vi "Shock&Dyanamics Laboratory - DROPBEAR_June2022_Rev3.vi"() -> ()   [LabVIEW 2019] (continued)
  in  "PF Card 1":dbl caption="Card" min=0.0 max=7.0 step=1.0 format="%0#2.1g"
  in  "PF Channel 1":dbl=1.0 caption="Channel" min=0.0 max=7.0 step=1.0 format="%0#2.1g"
  out "LED Enable Ch 1":bool=TRUE
  in  "SG Pair Ch 1":T10(ring)=enum."Ch 2"
  in  "SG Pair 2":bool caption="Paired"
  in  "Sens Fac 2":enum16{"uV/MU", "mV/MU", "V/MU"}(ring)=enum."mV/MU"
  in  "PF Condition 2":bool caption="PF Condition"
  in  "PF Chassis 2":dbl caption="Chassis" min=0.0 max=7.0 step=1.0 format="%0#2.1g"
  in  "PF Card 2":dbl caption="Card" min=0.0 max=7.0 step=1.0 format="%0#2.1g"
  in  "PF Channel 2":dbl caption="Channel" min=0.0 max=7.0 step=1.0 format="%0#2.1g"
  in  "Voltage Max Ch 2":dbl=10.0 caption="Max Value"
  in  "Voltage Min Ch 2":dbl=-10.0 caption="Min Value"
  in  "Enable Ch 2":bool=TRUE
  in  "Name Ch 2":string="SG_306_b"
  in  "Physical Channel Ch 2":tag="PXI1Slot5/ai1" caption="Physical Channels"
  in  "Sensitivity 2":dbl=50.0 caption="Sensitivity 0"
  out "LED Enable Ch 2":bool=TRUE
  in  "Signal Type 2":T8(ring)=enum."Strain" caption="Signal Type"
  in  "SG Pair Ch 2":T11(ring)=enum."Unpaired"
  in  "SG Pair 3":bool caption="Paired"
  in  "Sens Fac 3":enum16{"uV/MU", "mV/MU", "V/MU"}(ring)=enum."V/MU"
  in  "PF Condition 3":bool caption="PF Condition"
  in  "PF Chassis 3":dbl caption="Chassis" min=0.0 max=7.0 step=1.0 format="%0#2.1g"
  in  "PF Card 3":dbl caption="Card" min=0.0 max=7.0 step=1.0 format="%0#2.1g"
  in  "PF Channel 3":dbl=1.0 caption="Channel" min=0.0 max=7.0 step=1.0 format="%0#2.1g"
  in  "Voltage Max Ch 3":dbl=10.0 caption="Max Value"
  in  "Voltage Min Ch 3":dbl=-10.0 caption="Min Value"
  in  "Enable Ch 3":bool=TRUE
  in  "Name Ch 3":string="Accel"
  in  "Physical Channels Ch 3":tag="PXI1Slot5/ai4" caption="Physical Channels"
  in  "Sensitivity 3":dbl=2.0 caption="Sensitivity 0"
  out "LED Enable Ch 3":bool=TRUE
  in  "Signal Type 3":T8(ring) caption="Signal Type"
  in  "SG Pair Ch 3":T12(ring)=enum."Unpaired"
  in  "SG Pair 4":bool=TRUE caption="Paired"
  in  "Sens Fac 4":enum16{"uV/MU", "mV/MU", "V/MU"}(ring)=enum."mV/MU"
  in  "PF Condition 4":bool=TRUE caption="PF Condition"
  in  "PF Chassis 4":dbl caption="Chassis" min=0.0 max=7.0 step=1.0 format="%0#2.1g"
  in  "PF Card 4":dbl caption="Card" min=0.0 max=7.0 step=1.0 format="%0#2.1g"
  in  "PF Channel 4":dbl=2.0 caption="Channel" min=0.0 max=7.0 step=1.0 format="%0#2.1g"
  in  "Physical Channel Ch 4":tag="PXI1Slot5/ai5" caption="Physical Channels"
  in  "Name Ch 4":string="LowG_accel"
  in  "Enable Ch 4":bool
  in  "Voltage Max Ch 4":dbl=10.0 caption="Max Value"
  in  "Voltage Min Ch 4":dbl=-10.0 caption="Min Value"
  in  "Sensitivity 4":dbl=1.0 caption="Sensitivity 0"
  out "LED Enable Ch 4":bool
  in  "Signal Type 4":T8(ring)=enum."Voltage" caption="Signal Type"
  in  "SG Pair Ch 4":T13(ring)=enum."Unpaired"
  in  "SG Pair 5":bool=TRUE caption="Paired"
  in  "Sens Fac 5":enum16{"uV/MU", "mV/MU", "V/MU"}(ring)=enum."mV/MU"
  in  "Name Ch 5":string="MassDrop"
  in  "Physical Channel Ch 5":tag="PXI1Slot7/ai0" caption="Physical Channels"
  in  "Enable Ch 5":bool
  in  "Voltage Min Ch 5":dbl=-10.0 caption="Min Value"
  in  "Voltage Max Ch 5":dbl=10.0 caption="Max Value"
  in  "Sensitivity 5":dbl=1.0 caption="Sensitivity 0"
  out "LED Enable Ch 5":bool=TRUE
  in  "Signal Type 5":T8(ring)=enum."Voltage" caption="Signal Type"
  in  "PF Channel 5":dbl=3.0 caption="Channel" min=0.0 max=7.0 step=1.0 format="%0#2.1g"
  in  "PF Card 5":dbl caption="Card" min=0.0 max=7.0 step=1.0 format="%0#2.1g"
  in  "PF Chassis 5":dbl caption="Chassis" min=0.0 max=7.0 step=1.0 format="%0#2.1g"
  in  "PF Condition 5":bool=TRUE caption="PF Condition"
  in  "SG Pair Ch 5":T14(ring)=enum."Unpaired"
  in  "SG Pair 6":bool caption="Paired"
  in  "Sens Fac 6":enum16{"uV/MU", "mV/MU", "V/MU"}(ring)=enum."mV/MU"
  in  "Enable Ch 6":bool=TRUE
  in  "Physical Channels Ch 6":tag="PXI1Slot6/ai0" caption="Physical Channels"
  in  "Voltage Max  Ch 6":dbl=10.0 caption="Max Value"
  in  "Voltage Min Ch 6":dbl=-10.0 caption="Min Value"
  in  "Name Ch 6":string="PinLoc"
  in  "Sensitivity 6":dbl=1.0 caption="Sensitivity 0"
  out "LED Enable Ch 6":bool=TRUE
  in  "Signal Type 6":T8(ring)=enum."Voltage" caption="Signal Type"
  in  "PF Channel 6":dbl caption="Channel" min=0.0 max=7.0 step=1.0 format="%0#2.1g"
  in  "PF Card 6":dbl caption="Card" min=0.0 max=7.0 step=1.0 format="%0#2.1g"
  in  "PF Chassis 6":dbl caption="Chassis" min=0.0 max=7.0 step=1.0 format="%0#2.1g"
  in  "PF Condition 6":bool=TRUE caption="PF Condition"
  in  "SG Pair Ch 6":T15(ring)=enum."Unpaired"
  in  "SG Pair 7":bool=TRUE caption="Paired"
  in  "Sens Fac 7":enum16{"uV/MU", "mV/MU", "V/MU"}(ring)=enum."mV/MU"
  in  "PF Channel 7":dbl=1.0 caption="Channel" min=0.0 max=7.0 step=1.0 format="%0#2.1g"
  in  "PF Card 7":dbl caption="Card" min=0.0 max=7.0 step=1.0 format="%0#2.1g"
  in  "PF Chassis 7":dbl caption="Chassis" min=0.0 max=7.0 step=1.0 format="%0#2.1g"
  in  "PF Condition 7":bool=TRUE caption="PF Condition"
  in  "Enable Ch 7":bool=TRUE
  in  "Physical Channel Ch 7":tag="PXI1Slot7/ai3" caption="Physical Channels"
  in  "Voltage Max Ch 7":dbl=10.0 caption="Max Value"
  in  "Voltage Min Ch 7":dbl=-1.0 caption="Min Value"
  in  "Name Ch 7":string="Extensometer"
  in  "Sensitivity 7":dbl=1.0 caption="Sensitivity 0"
  out "LED Enable Ch 7":bool=TRUE
  in  "Signal Type 7":T8(ring)=enum."Voltage" caption="Signal Type"
  in  "SG Pair Ch 7":T16(ring)=enum."Unpaired"
  in  "SG Pair 8":bool=TRUE caption="Paired"
  in  "Sens Fac 8":enum16{"uV/MU", "mV/MU", "V/MU"}(ring)=enum."mV/MU"
  in  "Enable Ch 8":bool
  in  "Physical Channel Ch 8":tag="PXI1Slot7/ai2" caption="Physical Channels"
  in  "Voltage Max Ch 8":dbl=10.0 caption="Max Value"
  in  "Voltage Min Ch 8":dbl=-10.0 caption="Min Value"
  in  "Name Ch 8":string="StrainGauge_08_000"
  in  "Sensitivity 8":dbl=1.0 caption="Sensitivity 0"
  out "LED Enable Ch 8":bool
  in  "Signal Type 8":T8(ring)=enum."Strain" caption="Signal Type"
  in  "PF Condition 8":bool=TRUE caption="PF Condition"
  in  "PF Chassis 8":dbl caption="Chassis" min=0.0 max=7.0 step=1.0 format="%0#2.1g"
  in  "PF Card 8":dbl caption="Card" min=0.0 max=7.0 step=1.0 format="%0#2.1g"
  in  "PF Channel 8":dbl=2.0 caption="Channel" min=0.0 max=7.0 step=1.0 format="%0#2.1g"
  in  "SG Pair Ch 8":T17(ring)=enum."Unpaired"
  in  "SG Pair 9":bool=TRUE caption="Paired"
  in  "Sens Fac 9":enum16{"uV/MU", "mV/MU", "V/MU"}(ring)=enum."mV/MU"
  in  "PF Condition 9":bool=TRUE caption="PF Condition"
  in  "PF Chassis 9":dbl caption="Chassis" min=0.0 max=7.0 step=1.0 format="%0#2.1g"
  in  "PF Card 9":dbl caption="Card" min=0.0 max=7.0 step=1.0 format="%0#2.1g"
  in  "PF Channel 9":dbl=3.0 caption="Channel" min=0.0 max=7.0 step=1.0 format="%0#2.1g"
  in  "Enable Ch 9":bool
  in  "Physical Channel Ch 9":tag="PXI1Slot7/ai3" caption="Physical Channels"
  in  "Voltage Max Ch 9":dbl=10.0 caption="Max Value"
  in  "Voltage Min Ch 9":dbl=-10.0 caption="Min Value"
  in  "Name Ch 9":string="StrainGauge_08_180"
  in  "Sensitivity 9":dbl=1.0 caption="Sensitivity 0"
  out "LED Enable Ch 9":bool
  in  "Signal Type 9":T8(ring)=enum."Strain" caption="Signal Type"
  in  "SG Pair Ch 9":T18(ring)=enum."Unpaired"
  in  "SG Pair 10":bool=TRUE caption="Paired"
  in  "Sens Fac 10":enum16{"uV/MU", "mV/MU", "V/MU"}(ring)
  in  "PF Condition 10":bool caption="PF Condition"
  in  "PF Chassis 10":dbl caption="Chassis" min=0.0 max=7.0 step=1.0 format="%0#2.1g"
  in  "PF Card 10":dbl caption="Card" min=0.0 max=7.0 step=1.0 format="%0#2.1g"
  in  "PF Channel 10":dbl caption="Channel" min=0.0 max=7.0 step=1.0 format="%0#2.1g"
  in  "Enable Ch 10":bool
  in  "Physical Channel Ch 10":tag="PXI1Slot5/ai2" caption="Physical Channels"
  in  "Voltage Max Ch 10":dbl=10.0 caption="Max Value"
  in  "Voltage Min Ch 10":dbl=-10.0 caption="Min Value"
  in  "Name Ch 10":string="noname"
  in  "Sensitivity 10":dbl=0.2 caption="Sensitivity 0"
  out "LED Enable Ch 10":bool
  in  "Signal Type 10":T8(ring)=enum."Strain" caption="Signal Type"
  in  "SG Pair Ch 10":T19(ring)=enum."Unpaired"
  in  "SG Pair 11":bool=TRUE caption="Paired"
  in  "Sens Fac 11":enum16{"uV/MU", "mV/MU", "V/MU"}(ring)
  in  "PF Condition 11":bool caption="PF Condition"
  in  "PF Chassis 11":dbl caption="Chassis" min=0.0 max=7.0 step=1.0 format="%0#2.1g"
  in  "PF Card 11":dbl caption="Card" min=0.0 max=7.0 step=1.0 format="%0#2.1g"
  in  "PF Channel 11":dbl caption="Channel" min=0.0 max=7.0 step=1.0 format="%0#2.1g"
  in  "Enable Ch 11":bool
  in  "Physical Channel Ch 11":tag="PXI1Slot5/ai2" caption="Physical Channels"
  in  "Voltage Max Ch 11":dbl=10.0 caption="Max Value"
  in  "Voltage Min Ch 11":dbl=-10.0 caption="Min Value"
  in  "Name Ch 11":string="noname"
  in  "Sensitivity 11":dbl=0.2 caption="Sensitivity 0"
  out "LED Enable Ch 11":bool
  in  "Signal Type 11":T8(ring)=enum."Strain" caption="Signal Type"
  in  "SG Pair Ch 11":T20(ring)=enum."Unpaired"
  in  "SG Pair 12":bool=TRUE caption="Paired"
  in  "Sens Fac 12":enum16{"uV/MU", "mV/MU", "V/MU"}(ring)
  in  "PF Condition 12":bool caption="PF Condition"
  in  "PF Chassis 12":dbl caption="Chassis" min=0.0 max=7.0 step=1.0 format="%0#2.1g"
  in  "PF Card 12":dbl caption="Card" min=0.0 max=7.0 step=1.0 format="%0#2.1g"
  in  "PF Channel 12":dbl caption="Channel" min=0.0 max=7.0 step=1.0 format="%0#2.1g"
  in  "Enable Ch 12":bool
  in  "Physical Channel Ch 12":tag="PXI1Slot5/ai2" caption="Physical Channels"
  in  "Voltage Max Ch 12":dbl=10.0 caption="Max Value"
  in  "Voltage Min Ch 12":dbl=-10.0 caption="Min Value"
  in  "Name Ch 12":string="noname"
  in  "Sensitivity 12":dbl=0.2 caption="Sensitivity 0"
  out "LED Enable Ch 12":bool
  in  "Signal Type 12":T8(ring)=enum."Strain" caption="Signal Type"
  in  "SG Pair Ch 12":T21(ring)=enum."Unpaired"
  in  "SG Pair 13":bool=TRUE caption="Paired"
  in  "Sens Fac 13":enum16{"uV/MU", "mV/MU", "V/MU"}(ring)
  in  "PF Condition 13":bool caption="PF Condition"
  in  "PF Chassis 13":dbl caption="Chassis" min=0.0 max=7.0 step=1.0 format="%0#2.1g"
  in  "PF Card 13":dbl caption="Card" min=0.0 max=7.0 step=1.0 format="%0#2.1g"
  in  "PF Channel 13":dbl caption="Channel" min=0.0 max=7.0 step=1.0 format="%0#2.1g"
  in  "Enable Ch 13":bool
  in  "Physical Channel Ch 13":tag="PXI1Slot5/ai2" caption="Physical Channels"
  in  "Voltage Max Ch 13":dbl=10.0 caption="Max Value"
  in  "Voltage Min Ch 13":dbl=-10.0 caption="Min Value"
  in  "Name Ch 13":string="noname"
  in  "Sensitivity 13":dbl=0.2 caption="Sensitivity 0"
  out "LED Enable Ch 13":bool
  in  "Signal Type 13":T8(ring)=enum."Strain" caption="Signal Type"
  in  "SG Pair Ch 13":T22(ring)=enum."Unpaired"
  in  "SG Pair 14":bool=TRUE caption="Paired"
  in  "Sens Fac 14":enum16{"uV/MU", "mV/MU", "V/MU"}(ring)
  in  "PF Condition 14":bool caption="PF Condition"
  in  "PF Chassis 14":dbl caption="Chassis" min=0.0 max=7.0 step=1.0 format="%0#2.1g"
  in  "PF Card 14":dbl caption="Card" min=0.0 max=7.0 step=1.0 format="%0#2.1g"
  in  "PF Channel 14":dbl caption="Channel" min=0.0 max=7.0 step=1.0 format="%0#2.1g"
  in  "Enable Ch 14":bool
  in  "Physical Channel Ch 14":tag="PXI1Slot5/ai2" caption="Physical Channels"
  in  "Voltage Max Ch 14":dbl=10.0 caption="Max Value"
  in  "Voltage Min Ch 14":dbl=-10.0 caption="Min Value"
  in  "Name Ch 14":string="noname"
  in  "Sensitivity 14":dbl=0.2 caption="Sensitivity 0"
  out "LED Enable Ch 14":bool
  in  "Signal Type 14":T8(ring)=enum."Strain" caption="Signal Type"
  in  "SG Pair Ch 14":T23(ring)=enum."Unpaired"
  in  "SG Pair 15":bool=TRUE caption="Paired"
  in  "Sens Fac 15":enum16{"uV/MU", "mV/MU", "V/MU"}(ring)
  in  "PF Condition 15":bool caption="PF Condition"
  in  "PF Chassis 15":dbl caption="Chassis" min=0.0 max=7.0 step=1.0 format="%0#2.1g"
  in  "PF Card 15":dbl caption="Card" min=0.0 max=7.0 step=1.0 format="%0#2.1g"
  in  "PF Channel 15":dbl caption="Channel" min=0.0 max=7.0 step=1.0 format="%0#2.1g"
  in  "Enable Ch 15":bool
  in  "Physical Channel Ch 15":tag="PXI1Slot5/ai2" caption="Physical Channels"
  in  "Voltage Max Ch 15":dbl=10.0 caption="Max Value"
  in  "Voltage Min Ch 15":dbl=-10.0 caption="Min Value"
  in  "Name Ch 15":string="noname"
  in  "Sensitivity 15":dbl=0.2 caption="Sensitivity 0"
  out "LED Enable Ch 15":bool
  in  "Signal Type 15":T8(ring)=enum."Strain" caption="Signal Type"
  in  "SG Pair Ch 15":T24(ring)=enum."Unpaired"
  in  "Enable Ch 16":bool
  in  "Name Ch 16":string="noname"
  in  "Physical Channel Ch 16":tag="PXI1Slot8/ai3" caption="Physical Channels"
  in  "PF Chassis 16":dbl caption="Chassis" min=0.0 max=7.0 step=1.0 format="%0#2.1g"
  in  "PF Card 16":dbl=5.0 caption="Card" min=0.0 max=7.0 step=1.0 format="%0#2.1g"
  in  "PF Channel 16":dbl=3.0 caption="Channel" min=0.0 max=7.0 step=1.0 format="%0#2.1g"
  in  "PF Condition 16":bool=TRUE caption="PF Condition"
  in  "Signal Type 16":T8(ring)=enum."Strain" caption="Signal Type"
  in  "Voltage Max Ch 16":dbl=10.0 caption="Max Value"
  in  "Voltage Min Ch 16":dbl=-10.0 caption="Min Value"
  in  "Sensitivity 16":dbl=10.0 caption="Sensitivity 0"
  in  "Sens Fac 16":enum16{"uV/MU", "mV/MU", "V/MU"}(ring)=enum."mV/MU"
  in  "SG Pair 16":bool caption="Paired"
  out "LED Enable Ch 16":bool
  in  "SG Pair Ch 16":T25(ring)=enum."Unpaired"
  in  "Enable Ch 17":bool
  in  "Name Ch 17":string="noname"
  in  "Physical Channel Ch 17":tag="PXI1Slot5/ai2" caption="Physical Channels"
  in  "PF Channel 17":dbl caption="Channel" min=0.0 max=7.0 step=1.0 format="%0#2.1g"
  in  "PF Card 17":dbl caption="Card" min=0.0 max=7.0 step=1.0 format="%0#2.1g"
  in  "PF Chassis 17":dbl caption="Chassis" min=0.0 max=7.0 step=1.0 format="%0#2.1g"
  in  "PF Condition 17":bool caption="PF Condition"
  in  "Sensitivity 17":dbl=0.2 caption="Sensitivity 0"
  in  "Sens Fac 17":enum16{"uV/MU", "mV/MU", "V/MU"}(ring)
  in  "Signal Type 17":T8(ring)=enum."Strain" caption="Signal Type"
  in  "Voltage Max Ch 17":dbl=10.0 caption="Max Value"
  in  "Voltage Min Ch 17":dbl=-10.0 caption="Min Value"
  in  "SG Pair 17":bool=TRUE caption="Paired"
  out "LED Enable Ch 17":bool
  in  "SG Pair Ch 17":T26(ring)=enum."Unpaired"
  in  "Enable Ch 18":bool
  in  "Name Ch 18":string="noname"
  in  "Physical Channel Ch 18":tag="PXI1Slot5/ai2" caption="Physical Channels"
  in  "PF Channel 18":dbl caption="Channel" min=0.0 max=7.0 step=1.0 format="%0#2.1g"
  in  "PF Card 18":dbl caption="Card" min=0.0 max=7.0 step=1.0 format="%0#2.1g"
  in  "PF Chassis 18":dbl caption="Chassis" min=0.0 max=7.0 step=1.0 format="%0#2.1g"
  in  "PF Condition 18":bool caption="PF Condition"
  in  "Signal Type 18":T8(ring)=enum."Strain" caption="Signal Type"
  in  "Voltage Max Ch 18":dbl=10.0 caption="Max Value"
  in  "Voltage Min Ch 18":dbl=-10.0 caption="Min Value"
  in  "Sensitivity 18":dbl=0.2 caption="Sensitivity 0"
  in  "Sens Fac 18":enum16{"uV/MU", "mV/MU", "V/MU"}(ring)
  in  "SG Pair 18":bool=TRUE caption="Paired"
  out "LED Enable Ch 18":bool
  in  "SG Pair Ch 18":T27(ring)=enum."Unpaired"
  in  "Enable Ch 19":bool
  in  "Name Ch 19":string="noname"
  in  "Physical Channel Ch 19":tag="PXI1Slot5/ai2" caption="Physical Channels"
  in  "PF Channel 19":dbl caption="Channel" min=0.0 max=7.0 step=1.0 format="%0#2.1g"
  in  "PF Card 19":dbl caption="Card" min=0.0 max=7.0 step=1.0 format="%0#2.1g"
  in  "PF Chassis 19":dbl caption="Chassis" min=0.0 max=7.0 step=1.0 format="%0#2.1g"
  in  "PF Condition 19":bool caption="PF Condition"
  in  "Signal Type 19":T8(ring)=enum."Strain" caption="Signal Type"
  in  "Voltage Max Ch 19":dbl=10.0 caption="Max Value"
  in  "Voltage Min Ch 19":dbl=-10.0 caption="Min Value"
  in  "Sens Fac 19":enum16{"uV/MU", "mV/MU", "V/MU"}(ring)
  in  "Sensitivity 19":dbl=0.2 caption="Sensitivity 0"
  in  "SG Pair 19":bool=TRUE caption="Paired"
  out "LED Enable Ch 19":bool
  in  "SG Pair Ch 19":T28(ring)=enum."Unpaired"
  in  "Enable Ch 20":bool
  in  "Name Ch 20":string="noname"
  in  "Physical Channel Ch 20":tag="PXI1Slot5/ai2" caption="Physical Channels"
  in  "Voltage Max Ch 20":dbl=10.0 caption="Max Value"
  in  "Voltage Min Ch 20":dbl=-10.0 caption="Min Value"
  in  "Signal Type 20":T8(ring)=enum."Strain" caption="Signal Type"
  in  "Sensitivity 20":dbl=0.2 caption="Sensitivity 0"
  in  "Sens Fac 20":enum16{"uV/MU", "mV/MU", "V/MU"}(ring)
  in  "PF Chassis 20":dbl caption="Chassis" min=0.0 max=7.0 step=1.0 format="%0#2.1g"
  in  "PF Channel 20":dbl caption="Channel" min=0.0 max=7.0 step=1.0 format="%0#2.1g"
  in  "PF Card 20":dbl caption="Card" min=0.0 max=7.0 step=1.0 format="%0#2.1g"
  in  "PF Condition 20":bool caption="PF Condition"
  in  "SG Pair 20":bool=TRUE caption="Paired"
  out "LED Enable Ch 20":bool
  in  "SG Pair Ch 20":T29(ring)=enum."Unpaired"
  in  "Enable Ch 21":bool
  in  "Name Ch 21":string="noname"
  in  "Physical Channel Ch 21":tag="PXI1Slot5/ai2" caption="Physical Channels"
  in  "Voltage Max Ch 21":dbl=10.0 caption="Max Value"
  in  "Voltage Min Ch 21":dbl=-10.0 caption="Min Value"
  in  "PF Channel 21":dbl caption="Channel" min=0.0 max=7.0 step=1.0 format="%0#2.1g"
  in  "PF Card 21":dbl caption="Card" min=0.0 max=7.0 step=1.0 format="%0#2.1g"
  in  "PF Chassis 21":dbl caption="Chassis" min=0.0 max=7.0 step=1.0 format="%0#2.1g"
  in  "Sensitivity 21":dbl=0.2 caption="Sensitivity 0"
  in  "Sens Fac 21":enum16{"uV/MU", "mV/MU", "V/MU"}(ring)
  in  "PF Condition 21":bool caption="PF Condition"
  in  "Signal Type 21":T8(ring)=enum."Strain" caption="Signal Type"
  in  "SG Pair 21":bool=TRUE caption="Paired"
  out "LED Enable Ch 21":bool
  in  "SG Pair Ch 21":T30(ring)=enum."Unpaired"
  in  "Enable Ch 22":bool
  in  "Name Ch 22":string="noname"
  in  "Physical Channel Ch 22":tag="PXI1Slot5/ai2" caption="Physical Channels"
  in  "Sensitivity 22":dbl=0.2 caption="Sensitivity 0"
  in  "Signal Type 22":T8(ring)=enum."Strain" caption="Signal Type"
  in  "Sens Fac 22":enum16{"uV/MU", "mV/MU", "V/MU"}(ring)
  in  "PF Chassis 22":dbl caption="Chassis" min=0.0 max=7.0 step=1.0 format="%0#2.1g"
  in  "PF Card 22":dbl caption="Card" min=0.0 max=7.0 step=1.0 format="%0#2.1g"
  in  "PF Channel 22":dbl caption="Channel" min=0.0 max=7.0 step=1.0 format="%0#2.1g"
  in  "Voltage Max Ch 22":dbl=10.0 caption="Max Value"
  in  "Voltage Min Ch 22":dbl=-10.0 caption="Min Value"
  in  "PF Condition 22":bool caption="PF Condition"
  in  "SG Pair 22":bool caption="Paired"
  out "LED Enable Ch 22":bool
  in  "SG Pair Ch 22":T31(ring)=enum."Unpaired"
  in  "Enable Ch 23":bool
  in  "Name Ch 23":string="noname"
  in  "Physical Channel Ch 23":tag="PXI1Slot5/ai2" caption="Physical Channels"
  in  "Voltage Min Ch 23":dbl=-10.0 caption="Min Value"
  in  "Voltage Max Ch 23":dbl=10.0 caption="Max Value"
  in  "PF Channel 23":dbl caption="Channel" min=0.0 max=7.0 step=1.0 format="%0#2.1g"
  in  "PF Card 23":dbl caption="Card" min=0.0 max=7.0 step=1.0 format="%0#2.1g"
  in  "PF Chassis 23":dbl caption="Chassis" min=0.0 max=7.0 step=1.0 format="%0#2.1g"
  in  "Sens Fac 23":enum16{"uV/MU", "mV/MU", "V/MU"}(ring)
  in  "Sensitivity 23":dbl=0.2 caption="Sensitivity 0"
  in  "Signal Type 23":T8(ring)=enum."Strain" caption="Signal Type"
  in  "PF Condition 23":bool caption="PF Condition"
  in  "SG Pair 23":bool=TRUE caption="Paired"
  out "LED Enable Ch 23":bool
  in  "SG Pair Ch 23":T32(ring)=enum."Unpaired"
  in  "Enable Ch 24":bool
  in  "Name Ch 24":string="noname"
  in  "Physical Channel Ch 24":tag="PXI1Slot8/ai3" caption="Physical Channels"
  in  "Voltage Min Ch 24":dbl=-10.0 caption="Min Value"
  in  "Voltage Max Ch 24":dbl=10.0 caption="Max Value"
  in  "PF Chassis 24":dbl caption="Chassis" min=0.0 max=7.0 step=1.0 format="%0#2.1g"
  in  "PF Card 24":dbl=5.0 caption="Card" min=0.0 max=7.0 step=1.0 format="%0#2.1g"
  in  "PF Channel 24":dbl=3.0 caption="Channel" min=0.0 max=7.0 step=1.0 format="%0#2.1g"
  in  "PF Condition 24":bool=TRUE caption="PF Condition"
  in  "Signal Type 24":T8(ring)=enum."Strain" caption="Signal Type"
  in  "Sens Fac 24":enum16{"uV/MU", "mV/MU", "V/MU"}(ring)=enum."mV/MU"
  in  "Sensitivity 24":dbl=10.0 caption="Sensitivity 0"
  in  "SG Pair 24":bool=TRUE caption="Paired"
  out "LED Enable Ch 24":bool
  in  "SG Pair Ch 24":T33(ring)=enum."Unpaired"
  in  "Enable Ch 25":bool
  in  "Name Ch 25":string="noname"
  in  "Physical Channel Ch 25":tag="PXI1Slot5/ai2" caption="Physical Channels"
  in  "Voltage Min Ch 25":dbl=-10.0 caption="Min Value"
  in  "Voltage Max Ch 25":dbl=10.0 caption="Max Value"
  in  "PF Chassis 25":dbl caption="Chassis" min=0.0 max=7.0 step=1.0 format="%0#2.1g"
  in  "PF Card 25":dbl caption="Card" min=0.0 max=7.0 step=1.0 format="%0#2.1g"
  in  "PF Channel 25":dbl caption="Channel" min=0.0 max=7.0 step=1.0 format="%0#2.1g"
  in  "PF Condition 25":bool caption="PF Condition"
  in  "Sens Fac 25":enum16{"uV/MU", "mV/MU", "V/MU"}(ring)
  in  "Sensitivity 25":dbl=0.2 caption="Sensitivity 0"
  in  "Signal Type 25":T8(ring)=enum."Strain" caption="Signal Type"
  in  "SG Pair 25":bool=TRUE caption="Paired"
  out "LED Enable Ch 25":bool
  in  "SG Pair Ch 25":T34(ring)=enum."Unpaired"
  in  "Enable Ch 26":bool
  in  "Name Ch 26":string="noname"
  in  "Physical Channel Ch 26":tag="PXI1Slot5/ai2" caption="Physical Channels"
  in  "Sensitivity 26":dbl=0.2 caption="Sensitivity 0"
  in  "Sens Fac 26":enum16{"uV/MU", "mV/MU", "V/MU"}(ring)
  in  "PF Condition 26":bool caption="PF Condition"
  in  "PF Chassis 26":dbl caption="Chassis" min=0.0 max=7.0 step=1.0 format="%0#2.1g"
  in  "PF Card 26":dbl caption="Card" min=0.0 max=7.0 step=1.0 format="%0#2.1g"
  in  "PF Channel 26":dbl caption="Channel" min=0.0 max=7.0 step=1.0 format="%0#2.1g"
  in  "Voltage Min Ch 26":dbl=-10.0 caption="Min Value"
  in  "Voltage Max Ch 26":dbl=10.0 caption="Max Value"
  in  "Signal Type 26":T8(ring)=enum."Strain" caption="Signal Type"
  in  "SG Pair 26":bool=TRUE caption="Paired"
  out "LED Enable Ch 26":bool
  in  "SG Pair Ch 26":T35(ring)=enum."Unpaired"
  in  "Enable Ch 27":bool
  in  "Name Ch 27":string="noname"
  in  "Physical Channel Ch 27":tag="PXI1Slot5/ai2" caption="Physical Channels"
  in  "PF Chassis 27":dbl caption="Chassis" min=0.0 max=7.0 step=1.0 format="%0#2.1g"
  in  "PF Card 27":dbl caption="Card" min=0.0 max=7.0 step=1.0 format="%0#2.1g"
  in  "PF Channel 27":dbl caption="Channel" min=0.0 max=7.0 step=1.0 format="%0#2.1g"
  in  "PF Condition 27":bool caption="PF Condition"
  in  "Sensitivity 27":dbl=0.2 caption="Sensitivity 0"
  in  "Sens Fac 27":enum16{"uV/MU", "mV/MU", "V/MU"}(ring)
  in  "Signal Type 27":T8(ring)=enum."Strain" caption="Signal Type"
  in  "Voltage Max Ch 27":dbl=10.0 caption="Max Value"
  in  "Voltage Min Ch 27":dbl=-10.0 caption="Min Value"
  in  "SG Pair 27":bool=TRUE caption="Paired"
  out "LED Enable Ch 27":bool
  in  "SG Pair Ch 27":T36(ring)=enum."Unpaired"
  in  "Enable Ch 28":bool
  in  "Name Ch 28":string="noname"
  in  "Physical Channel Ch 28":tag="PXI1Slot5/ai2" caption="Physical Channels"
  in  "Sensitivity 28":dbl=0.2 caption="Sensitivity 0"
  in  "Sens Fac 28":enum16{"uV/MU", "mV/MU", "V/MU"}(ring)
  in  "Signal Type 28":T8(ring)=enum."Strain" caption="Signal Type"
  in  "PF Chassis 28":dbl caption="Chassis" min=0.0 max=7.0 step=1.0 format="%0#2.1g"
  in  "PF Card 28":dbl caption="Card" min=0.0 max=7.0 step=1.0 format="%0#2.1g"
  in  "PF Channel 28":dbl caption="Channel" min=0.0 max=7.0 step=1.0 format="%0#2.1g"
  in  "PF Condition 28":bool caption="PF Condition"
  in  "Voltage Min Ch 28":dbl=-10.0 caption="Min Value"
  in  "Voltage Max Ch 28":dbl=10.0 caption="Max Value"
  in  "SG Pair 28":bool=TRUE caption="Paired"
  out "LED Enable Ch 28":bool
  in  "SG Pair Ch 28":T37(ring)=enum."Unpaired"
  in  "Enable Ch 29":bool
  in  "Name Ch 29":string="noname"
  in  "Physical Channel Ch 29":tag="PXI1Slot5/ai2" caption="Physical Channels"
  in  "Signal Type 29":T8(ring)=enum."Strain" caption="Signal Type"
  in  "PF Chassis 29":dbl caption="Chassis" min=0.0 max=7.0 step=1.0 format="%0#2.1g"
  in  "PF Card 29":dbl caption="Card" min=0.0 max=7.0 step=1.0 format="%0#2.1g"
  in  "PF Channel 29":dbl caption="Channel" min=0.0 max=7.0 step=1.0 format="%0#2.1g"
  in  "PF Condition 29":bool caption="PF Condition"
  in  "Voltage Max Ch 29":dbl=10.0 caption="Max Value"
  in  "Voltage Min Ch 29":dbl=-10.0 caption="Min Value"
  in  "Sens Fac 29":enum16{"uV/MU", "mV/MU", "V/MU"}(ring)
  in  "Sensitivity 29":dbl=0.2 caption="Sensitivity 0"
  in  "SG Pair 29":bool caption="Paired"
  out "LED Enable Ch 29":bool
  in  "SG Pair Ch 29":T38(ring)=enum."Unpaired"
  in  "Enable Ch 30":bool
  in  "Name Ch 30":string="noname"
  in  "Physical Channel Ch 30":tag="PXI1Slot5/ai2" caption="Physical Channels"
  in  "Voltage Min Ch 30":dbl=-10.0 caption="Min Value"
  in  "Signal Type 30":T8(ring)=enum."Strain" caption="Signal Type"
  in  "Voltage Max Ch 30":dbl=10.0 caption="Max Value"
  in  "Sensitivity 30":dbl=0.2 caption="Sensitivity 0"
  in  "Sens Fac 30":enum16{"uV/MU", "mV/MU", "V/MU"}(ring)
  in  "PF Chassis 30":dbl caption="Chassis" min=0.0 max=7.0 step=1.0 format="%0#2.1g"
  in  "PF Card 30":dbl caption="Card" min=0.0 max=7.0 step=1.0 format="%0#2.1g"
  in  "PF Channel 30":dbl caption="Channel" min=0.0 max=7.0 step=1.0 format="%0#2.1g"
  in  "PF Condition 30":bool caption="PF Condition"
  in  "SG Pair 30":bool=TRUE caption="Paired"
  out "LED Enable Ch 30":bool
  in  "SG Pair Ch 30":T39(ring)=enum."Unpaired"
  in  "Enable Ch 31":bool
  in  "Name Ch 31":string="noname"
  in  "Physical Channel Ch 31":tag="PXI1Slot5/ai2" caption="Physical Channels"
  in  "Voltage Min Ch 31":dbl=-10.0 caption="Min Value"
  in  "Voltage Max Ch 31":dbl=10.0 caption="Max Value"
  in  "PF Chassis 31":dbl caption="Chassis" min=0.0 max=7.0 step=1.0 format="%0#2.1g"
  in  "PF Card 31":dbl caption="Card" min=0.0 max=7.0 step=1.0 format="%0#2.1g"
  in  "PF Channel 31":dbl caption="Channel" min=0.0 max=7.0 step=1.0 format="%0#2.1g"
  in  "Sensitivity 31":dbl=0.2 caption="Sensitivity 0"
  in  "Sens Fac 31":enum16{"uV/MU", "mV/MU", "V/MU"}(ring)
  in  "Signal Type 31":T8(ring)=enum."Strain" caption="Signal Type"
  in  "PF Condition 31":bool caption="PF Condition"
  in  "SG Pair 31":bool=TRUE caption="Paired"
  out "LED Enable Ch 31":bool
  in  "SG Pair Ch 31":T40(ring)=enum."Unpaired"
  out "Instructions":string="Specify directory and file name for log file. Labview will automatically append date and time stamp to file name after every test if Enable Data Logging is set to \"True\"."
  in  "Folder Name to Save Raw Data":string="C:\\Users\\PXIe-8880\\Desktop\\Projects\\DROPBEAR\\Practice\\"
  in  "File Name to Save Raw Data":string="test1.txt"
  in  "?":bool
  in  "Separated":bool
  in  "?":bool
  out "?":bool=TRUE
  in  "First Pulse":bool
  in  "Incident Name for First Pulse\n(Must Match Exactly":string
  # "Extensometer Settings"
  # "Extensometer Readings"
  # "Acquired Data"
  # "Longitudinal Strain"
  # "Bending Strain"
  # "Velocity"
  # "Acceleration"
  # "Precision Filters Information"
  # "Precision Filters Information"
  # "Precision Filters Information"
  # "Precision Filters Information"
  # "Precision Filters Information"
  # "Precision Filters Information"
  # "Precision Filters Information"
  # "Precision Filters Information"
  # "Precision Filters Information"
  # "Precision Filters Information"
  # "Precision Filters Information"
  # "Precision Filters Information"
  # "Precision Filters Information"
  # "Precision Filters Information"
  # "Precision Filters Information"
  # "Precision Filters Information"
  # "Precision Filters Information"
  # "Precision Filters Information"
  # "Precision Filters Information"
  # "Precision Filters Information"
  # "Precision Filters Information"
  # "Precision Filters Information"
  # "Precision Filters Information"
  # "Precision Filters Information"
  # "Precision Filters Information"
  # "Precision Filters Information"
  # "Precision Filters Information"
  # "Precision Filters Information"
  # "Precision Filters Information"
  # "Precision Filters Information"
  # "Precision Filters Information"
  # "Precision Filters Information"
  # "Channel Settings"
  # "Timing/Trigger"
